vi "Create_Trajectory_Using_PathfinderDifferential_ORIG.vi"() -> ()   [LabVIEW 2019]
uses:
  <vilib>/Rock Robotics/WPI/ThirdParty/JAS_Junk/JaciPathFinderLib/VIs/Waypoint.ctl
  <vilib>/Rock Robotics/WPI/ThirdParty/JAS_Junk/TrajLib/TRAJ_STATE.ctl
  <vilib>/Rock Robotics/WPI/ThirdParty/JAS_Junk/TrajLib/POSE2D.ctl
  <vilib>/Rock Robotics/WPI/ThirdParty/JAS_Junk/TrajLib/TRANSLATION2D.ctl
  <vilib>/Rock Robotics/WPI/ThirdParty/JAS_Junk/TrajLib/ROTATION2D.ctl
  <vilib>/Rock Robotics/WPI/ThirdParty/JAS_Junk/TrajLib/UTIL_PATHFINDER_CONFIG.ctl
  <vilib>/Rock Robotics/WPI/ThirdParty/JAS_Junk/TrajLib/DISPLAY_WAYPOINT.ctl
  <vilib>/Rock Robotics/WPI/ThirdParty/JAS_Junk/JaciPathFinderLib/Pathfinder.lvlib
  <vilib>/Rock Robotics/WPI/ThirdParty/JAS_Junk/TrajLib/Trajectory_Library.lvlib
panel:
  in  "End Program":bool
  in  "Tab Control":T1(tab)
  in  "max_velocity":dbl=58.0
  in  "max_acceleration":dbl=65.0
  in  "max_jerk":dbl=70.0
  in  "wheelbase_width":dbl=20.866
  in  "Real max\n speed":dbl=65.0
  out "max speed":dbl
  out "Path \nSpeed > \nMax":bool
  out "Complete,\nReady to \nSave file":bool
  in  "Calculate\nPath":bool
  out "Path calculation error":errorcluster
  in  "sample_count":i32=100000
  in  "Path Results\ndT":dbl=0.02 format="%7.3f"
  in  "?":T2[](array[typedef])=[{"x"=15.0, "y"=105.0, "angle"=-45.0}, {"x"=105.0, "y"=65.0, "angle"=0.0}, {"x"=210.0, "y"=106.0, "angle"=45.0}]
  out "Position":cluster{dbl[], dbl[]}[](graph)
  out "Path Data":cluster{dbl[], dbl[]}[](graph)
  out "Traj States\nSize":i32
  out "Trajectory States":T3[](array[typedef]) {"POSE"."ROTATION"."SIN" format="%13.4f"; "POSE"."ROTATION"."COS" format="%13.4f"; "POSE"."ROTATION"."VALUE" format="%13.4f"; "POSE"."TRANSLATION"."Y" format="%14.3f"; "POSE"."TRANSLATION"."X" format="%14.3f"}
  out "File Saved\nWithout\nError":bool
  in  "Trajectory Type":enum32{"Radio Selection 1", "Radio Selection 2"}(radio)
  out "File Creation\nError":errorcluster
  in  "Trajectory File Comment":string
  in  "Trajectory File Name":path
  in  "CreateCmdList":bool
  # "Create trajectory using \"Jaci's Pathfinder\"  (Display for differential drive robot)"
  # "Instructions:\n----------------  \nThis utility will create a trajectory,, show the data on the various tabs, and optionally write a \"robot relative\" trajectory to a \nfile. To use this utility:\n\n1) Read all of these instructions!\n2) Define the Robot Data. on the \"Robot Data\" tab.\n3) Define the \"Path Definition\" on the \"Define / Create Trajectory\" tab.  These are the beginning and ending positions/headings, and \n     internal positions/headings.\n4) Define the time increment.  0.020 is chosen since that matches the normal robot loop time.\n5) Define \"sample count\".  This is an internal PathFinder variable.  Leaving the value as default should work correctly.  Making \n    the value a little smaller will speed the program up a little.\n6) Press the \"Calculate Path\".  If a good path was calculated it will be displayed on the \"Field Position tab, and the \"Complete, \n    Ready to Save\" indicator will light.  The path can be recalculated many times before performing any other action.\n\nAfter a Path has been calculated, the \"trajectory can be written to a file.  The absolute path is converted to a robot relative \ntrajectory.  To do this:\n1) Enter a comment to be included in the file.  Anything can be entered.\n2) Select the file name.\n3) Select the type of trajectory to save, absolute or relative.\n4) Press \"Create Trajectory File\"  If an error occurs it will be displayed in the File Creation Error indicator.\n\nNotes:\n---------\n- All the robot parameters, path, and field dimensions are in INCHES, and DEGREES.  The resulting trajectory is converted to \n   METERS, and RADIANS to match the rest of this library!\n- The pathfinder path generation logic doesn't account distribution of speed to the left and right wheels.  As a result the \n   maximum speed can be exceeded.If this happens, but Path Speed > Max light will light and Ready to Execute will not \n   light.  Lower the maximum speed in the Robot Data tab and recalulate the path.  (CURRENTLY THIS LOGIC IS NOT COMPLETE.)\n- 2019 playing field size - width: 26 ft 11.25 In = 323.25 in , length: 52 ft 5.25 in = 629.25 in  (I didn't verify this for the 2020 version.)"
  # "ROBOT DATA"
  # "INCHES/SEC"
  # "INCHES/SEC"
  # "INCHES/SEC^2"
  # "INCHES/SEC^3"
  # "Simulated robot wheelbase is: 20.866"
  # "INCHES"
  # "Simulated robot max speed is: 68.266"
  # "PATH DEFINITION"
  # "SEC"
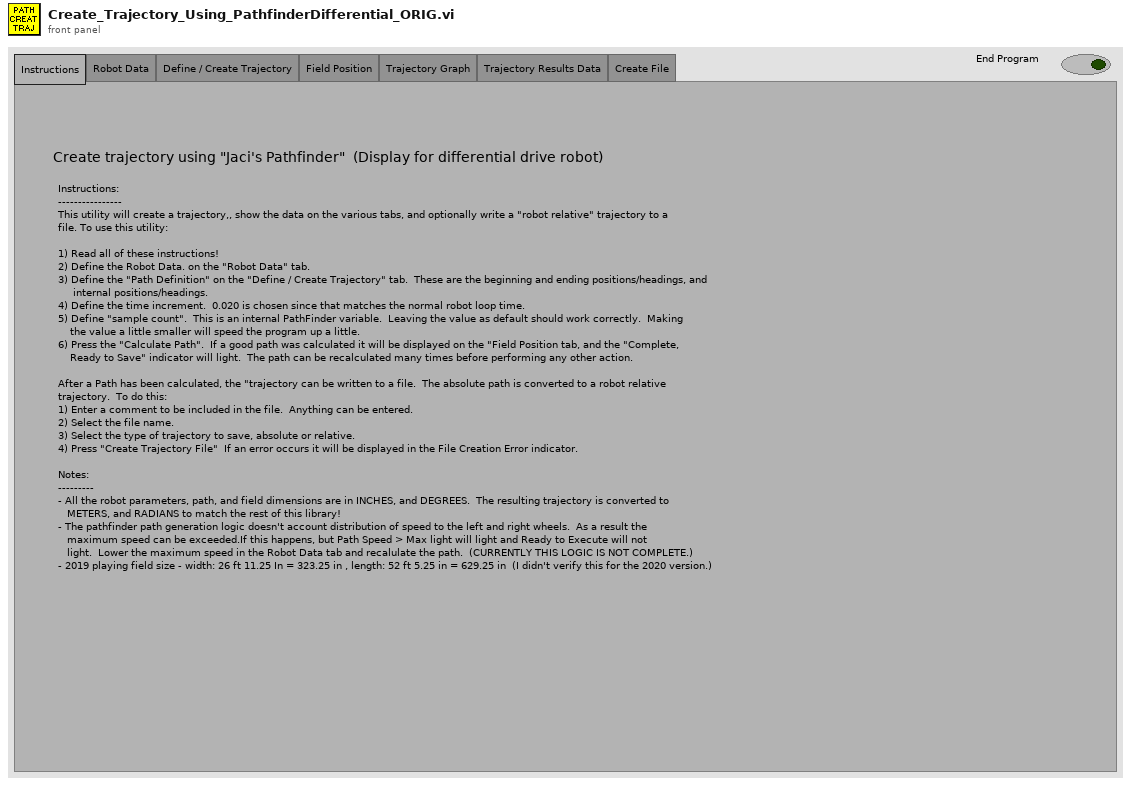
[diagram p1: front panel]
types:
  T1 = enum32{"Instructions", "Robot Data", "Define / Create Trajectory", "Field Position", "Trajectory Graph", "Trajectory Results Data", "Create File"}
  T2 = typedef "Pathfinder.lvlib/Waypoint.ctl" = cluster{"x":dbl, "y":dbl, "angle":dbl}
  T3 = typedef "Trajectory_Library.lvlib/TRAJ_STATE.ctl" = cluster{"TimeSeconds":dbl, "Velocity":dbl, "Acceleration":dbl, "POSE":T4, "Curvature":dbl}
  T4 = typedef "Trajectory_Library.lvlib/POSE2D.ctl" = cluster{"TRANSLATION":T5, "ROTATION":T6}
  T5 = typedef "Trajectory_Library.lvlib/TRANSLATION2D.ctl" = cluster{"X":dbl, "Y":dbl}
  T6 = typedef "Trajectory_Library.lvlib/ROTATION2D.ctl" = cluster{"VALUE":dbl, "COS":dbl, "SIN":dbl}
  T7 = typedef "Trajectory_Library.lvlib/DISPLAY_WAYPOINT.ctl" = cluster{"X":dbl, "Y":dbl, "ANGLE":dbl}
  T8 = typedef "Trajectory_Library.lvlib/UTIL_PATHFINDER_CONFIG.ctl" = cluster{"PathfinderType - 0 tank 1 serve":i32, "PathMaxVelocity - inches per sec":dbl, "MaxAcceleration - inches per sec2":dbl, "MaxJerk--Inches per sec2":dbl, "TimeDelta-Seconds":dbl, "SampleCount":i32, "WheelbaseWidth-inches":dbl, "WheelbaseDepth-inches":dbl, "SwerveType":i32, "ActualMaxVelocity-inches per sec":dbl}
  T9 = typedef "Trajectory_Library.lvlib/TRAJECTORY.ctl" = cluster{"TotalTImeSecs":dbl, "States":T3[]}
  T10 = typedef "Pathfinder.lvlib/Segment.ctl" = cluster{"dt":dbl, "x":dbl, "y":dbl, "position":dbl, "velocity":dbl, "acceleration":dbl, "jerk":dbl, "heading":dbl}
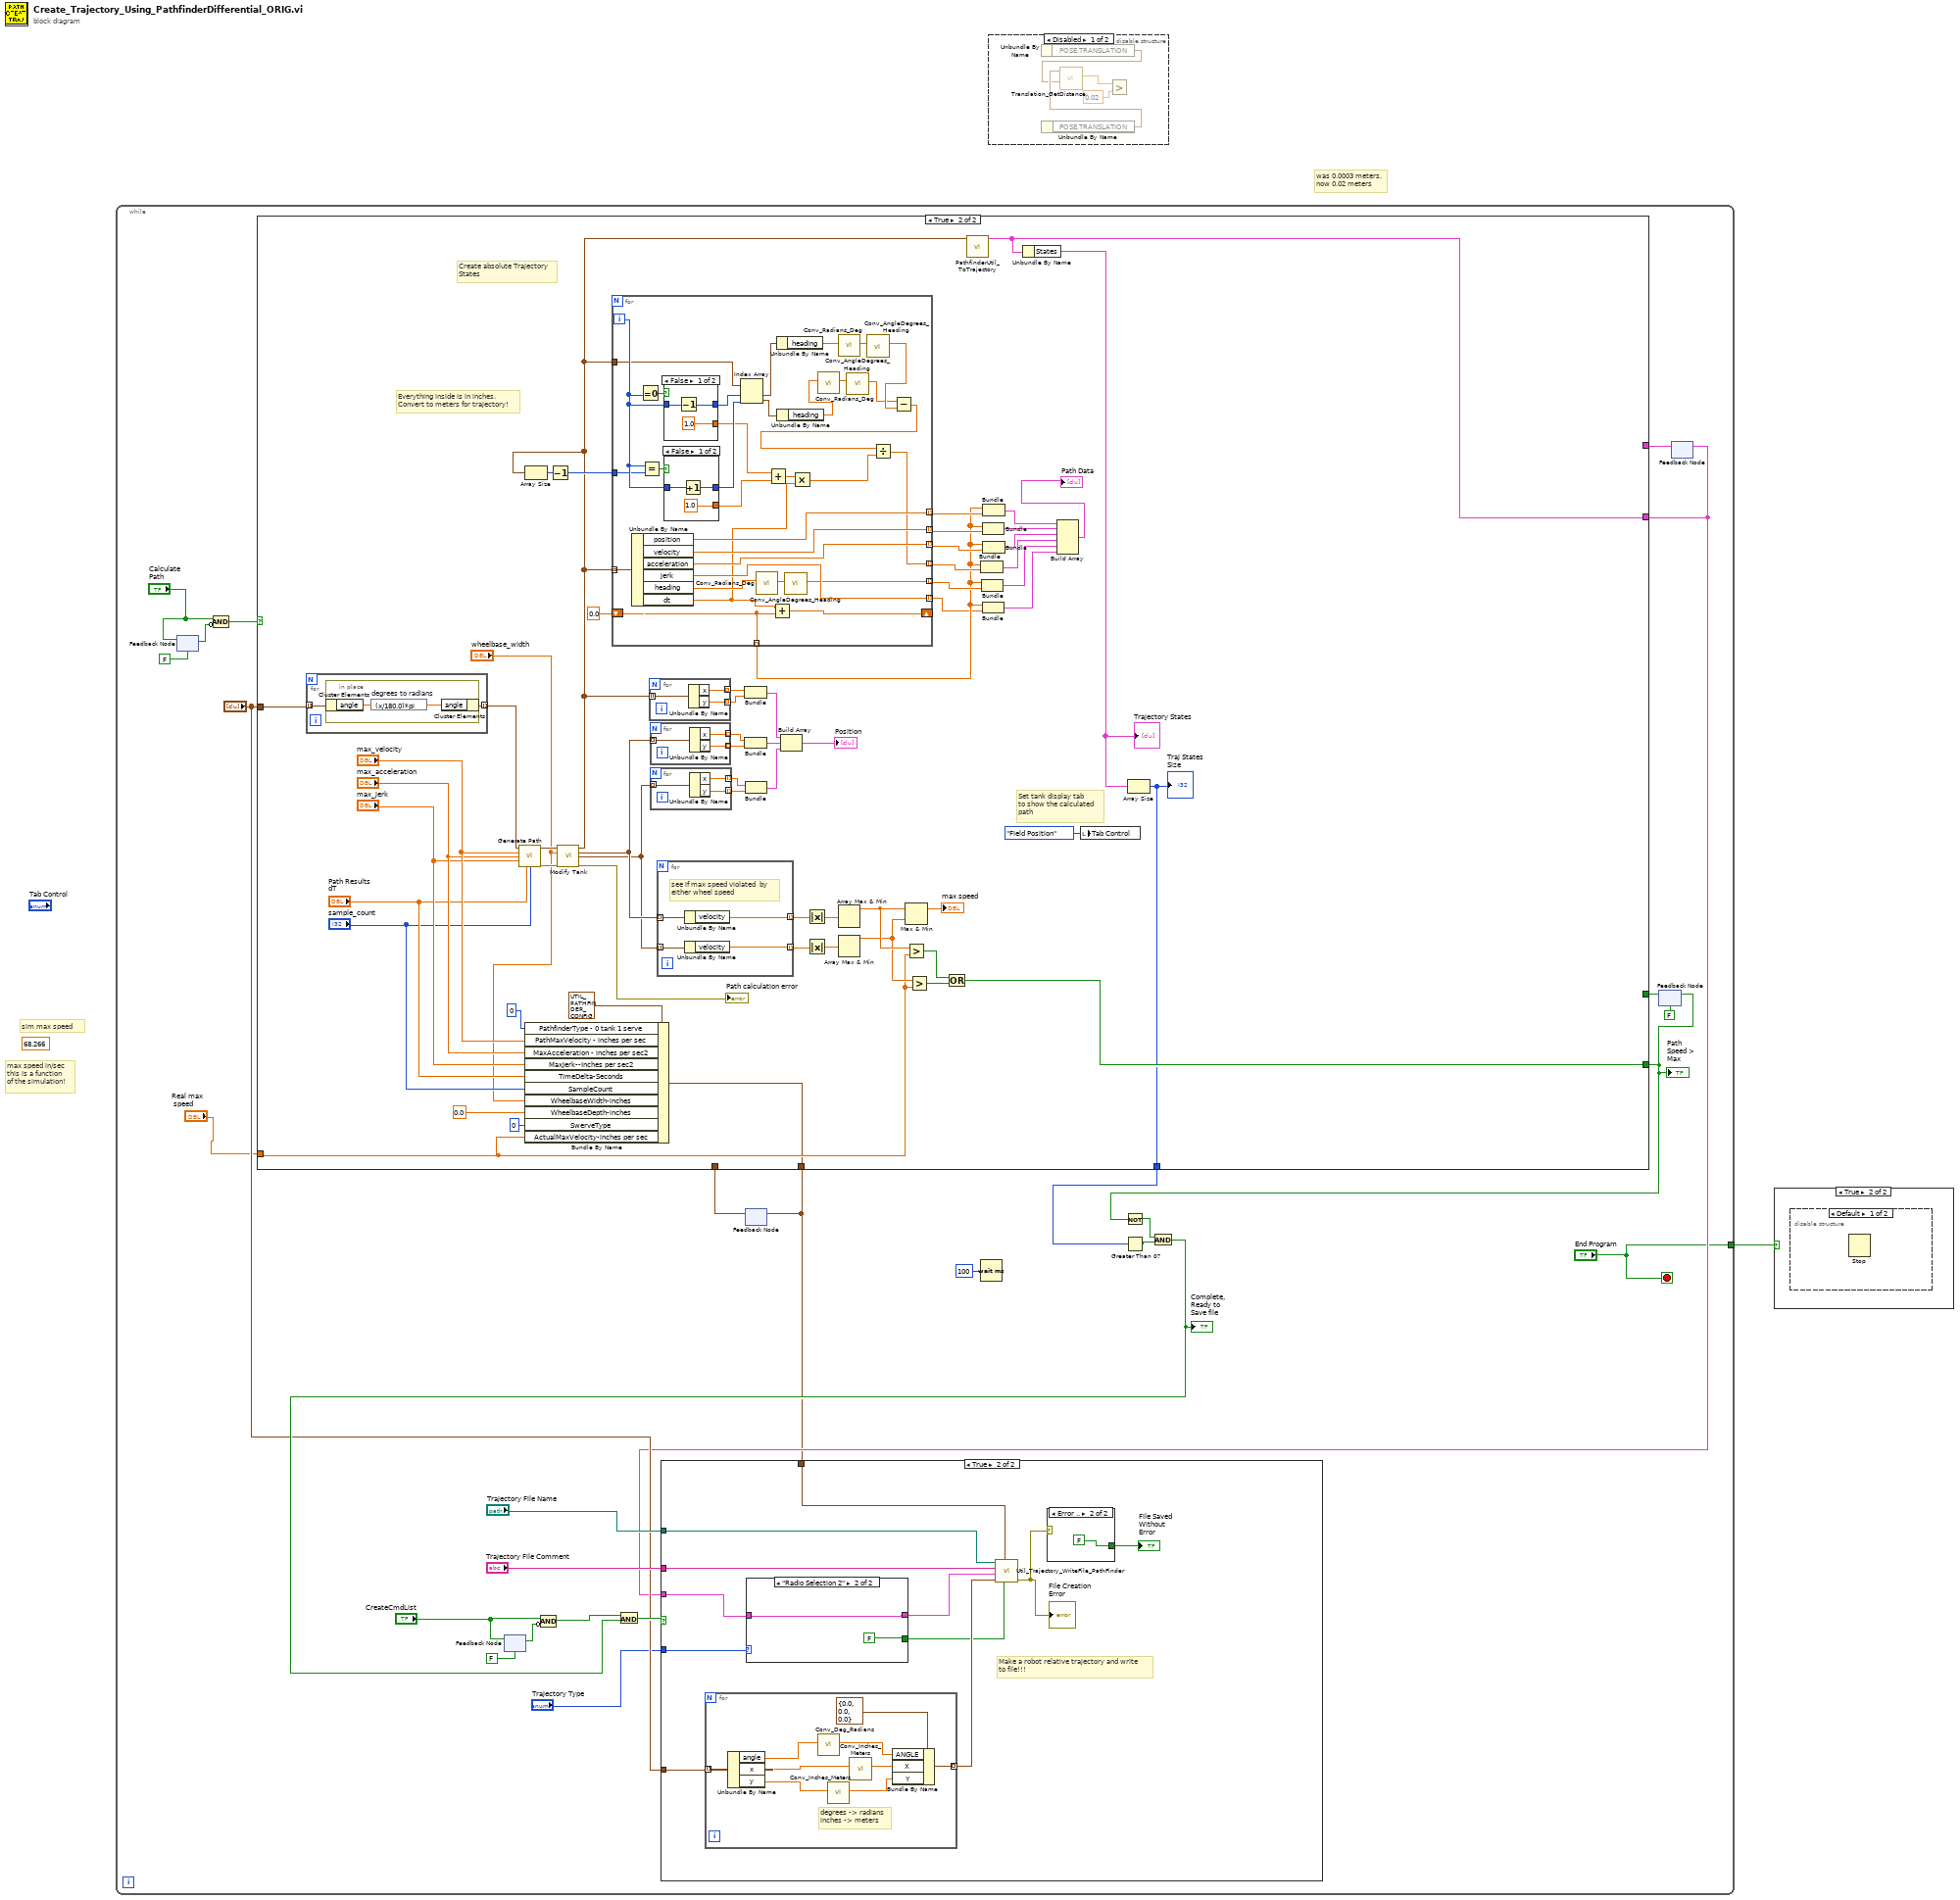
[diagram p0: block diagram]
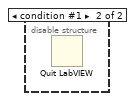
[diagram p3: hidden frame]
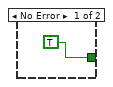
[diagram p6: hidden frame]
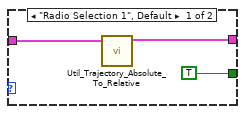
[diagram p7: hidden frame]
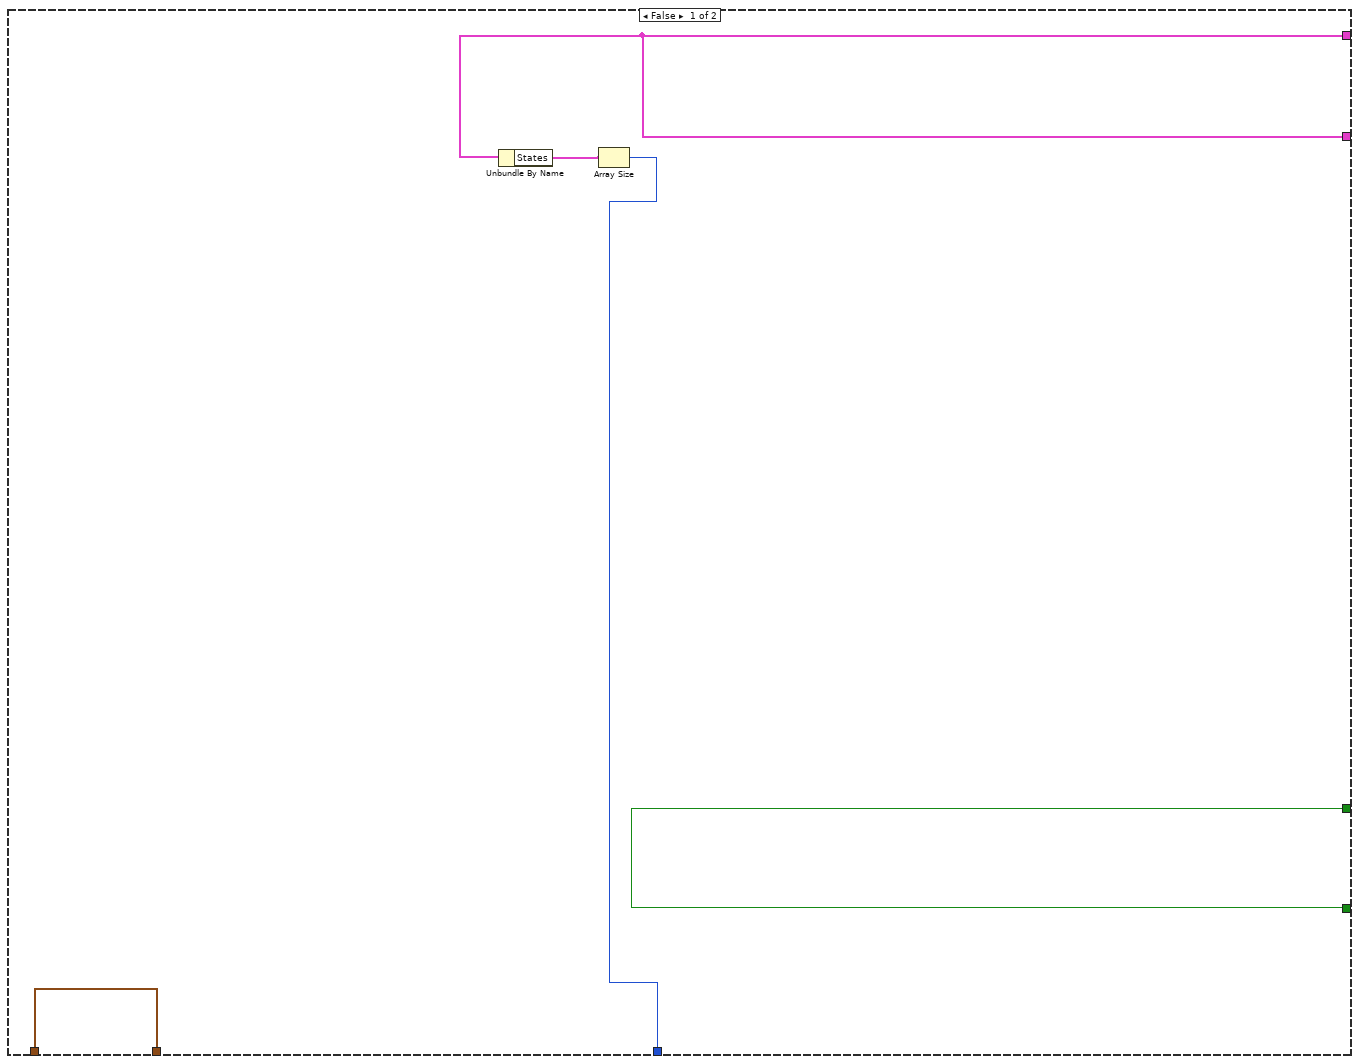
[diagram p8: hidden frame]
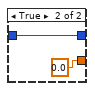
[diagram p9: hidden frame]
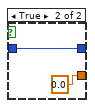
[diagram p10: hidden frame]
diagram:
  (unwired) 68.266 ("x")
  # "was 0.0003 meters.\nnow 0.02 meters"
  # "sim max speed"
  # "max speed in/sec\nthis is a function\nof the simulation!"
  n1 = while {
    tunnel: ["End Program"] -> w1
    stop <- "End Program" stop-if-true
    n2 = feedback #1(FALSE ("CreateCmdList")) -> (w10:bool)
    n3 = feedback-in #1("Calculate\nPath") -> ()
    n4 = Compound Arithmetic op=AND("Calculate\nPath", invert w10) -> (w7:bool)
    n5 = feedback-in #2("CreateCmdList") -> ()
    n6 = feedback #2(FALSE ("CreateCmdList")) -> (w13:bool)
    n7 = Compound Arithmetic op=AND("CreateCmdList", invert w13) -> (w12:bool)
    n8 = feedback #3() -> (w2:T8)  [unwired: 1 in]
    n9 = Wait (ms)(milliseconds to wait=u32 100) -> ()  [unwired: 1 out]
    n10 = feedback #4(FALSE) -> (w26:bool)
    n11 = feedback #5() -> (w22:T9)  [unwired: 1 in]
    n12 = case shown="True" w7 {
      tunnel: "Real max\n speed" -> [_ w65]
      tunnel: [w60 w106] -> w23
      tunnel: w26 -> [w60 _]
      tunnel: "?" -> [_ w105]
      tunnel: [w57 w82] -> w16
      tunnel: w22 -> [w57 _]
      tunnel: [w59 w97] -> w15
      tunnel: [w56 w61] -> w3
      tunnel: w2 -> [w56 _]
      frame False {
        n13 = Unbundle By Name(w57) -> ("States"=w58:T3[])
        n14 = Array Size(array=w58) -> (size(s)=w59:i32)
      }
      frame True {
        # "Everything inside is in inches.\nConvert to meters for trajectory!"
        # "Create absolute Trajectory\nStates"
        # "Set tank display tab\nto show the calculated\npath"
        n15 = for {
          tunnel: w105 -> [w127] mode=indexing
          tunnel: [w126] -> w119 mode=indexing
          n16 = in-place {
            n17 = in-place-cluster #6(w127) -> ("angle"=w129:dbl)
            n18 = expression code="(x/180.0)*pi" "degrees to radians"(w129) -> (w128:dbl)
            n19 = in-place-cluster #6("angle"=w128) -> (w126:T2)
          }
        }
        n20 = call <vilib>:"Generate Path.vi"("path"=w119, "max_velocity"="max_velocity", "max_acceleration"="max_acceleration", "max_jerk"="max_jerk", "dt (.001)"="Path Results\ndT", "sample_count (100000)"="sample_count") -> ("Segments"=w120:T10[], "error out"=w109:errorcluster)  [unwired: 8 in]
        n21 = Bundle By Name(cluster=T8 {"PathfinderType - 0 tank 1 serve"=0, "PathMaxVelocity - inches per sec"=0.0, "MaxAcceleration - inches per sec2"=0.0, "MaxJerk--Inches per sec2"=0.0, "TimeDelta-Seconds"=0.0, "SampleCount"=0, "WheelbaseWidth-inches"=0.0, "WheelbaseDepth-inches"=0.0, "SwerveType"=0, "ActualMaxVelocity-inches per sec"=0.0} ("UTIL_PATHFINDER_CONFIG"), "PathfinderType - 0 tank 1 serve"=0, "PathMaxVelocity - inches per sec"="max_velocity", "MaxAcceleration - inches per sec2"="max_acceleration", "MaxJerk--Inches per sec2"="max_jerk", "TimeDelta-Seconds"="Path Results\ndT", "SampleCount"="sample_count", "WheelbaseWidth-inches"="wheelbase_width", "WheelbaseDepth-inches"=0.0, "SwerveType"=0, "ActualMaxVelocity-inches per sec"=w65) -> (w61:T8)
        n22 = call <vilib>:"Modify Tank.vi"("Original"=w120, "wheelbase_width"="wheelbase_width", "error in"=w109) -> ("original"=w73:T10[], "left"=w104:T10[], "right"=w103:T10[], "error out"=→"Path calculation error":errorcluster)  [unwired: 9 in]
        n23 = Array Size(array=w73) -> (size(s)=w75:i32)
        n24 = Decrement(x=w75) -> (x-1=w74:i32)
        n25 = for {
          tunnel: w73 -> [w170] mode=indexing
          shift-right: [w168] -> _
          shift-left: 0.0 -> [w169]
          tunnel: [w169] -> w78 mode=indexing
          tunnel: [w161] -> w79 mode=indexing
          tunnel: [w167] -> w77 mode=indexing
          tunnel: [w166] -> w87 mode=indexing
          tunnel: [w165] -> w86 mode=indexing
          tunnel: [w164] -> w81 mode=indexing
          tunnel: [w147] -> w80 mode=indexing
          tunnel: w73 -> [w153]
          tunnel: w74 -> [w146]
          i -> [w158]
          n26 = Unbundle By Name(w170) -> ("position"=w164:dbl, "velocity"=w165:dbl, "acceleration"=w166:dbl, "jerk"=w167:dbl, "heading"=w163:dbl, "dt"=w149:dbl)
          n27 = Equal To 0?(x=w158) -> (x = 0?=w160:bool)
          n28 = Equal?(x=w158, y=w146) -> (x = y?=w159:bool)
          n29 = case shown="False" w160 {
            tunnel: w158 -> [w178 w179]
            tunnel: [1.0 0.0] -> w150
            tunnel: [w176 w179] -> w155
            frame False {
              n30 = Decrement(x=w178) -> (x-1=w176:i32)
            }
            frame True {
            }
          }
          n31 = case shown="False" w159 {
            tunnel: [1.0 0.0] -> w151
            tunnel: w158 -> [w172 w174]
            tunnel: [w171 w174] -> w154
            frame False {
              n32 = Increment(x=w172) -> (x+1=w171:i32)
            }
            frame True {
            }
          }
          n33 = Index Array(array=w153, index #1=w155, index #2=w154) -> (element #1=w157:T10, element #2=w156:T10)
          n34 = call <vilib>:"Conv_Radians_Deg.vi"("Radians"=w163) -> ("Degrees"=w162:dbl)  [unwired: 10 in]
          n35 = Add(x=w150, y=w151) -> (x+y=w152:dbl)
          n36 = Add(x=w149, y=w169) -> (x+y=w168:dbl)
          n37 = Unbundle By Name(w157) -> ("heading"=w143:dbl)
          n38 = Unbundle By Name(w156) -> ("heading"=w141:dbl)
          n39 = call <vilib>:"Conv_AngleDegrees_Heading.vi"("Degrees"=w162) -> ("Heading Degrees"=w161:dbl)  [unwired: 10 in]
          n40 = Multiply(x=w152, y=w149) -> (x*y=w148:dbl)
          n41 = call <vilib>:"Conv_Radians_Deg.vi"("Radians"=w141) -> ("Degrees"=w140:dbl)  [unwired: 10 in]
          n42 = call <vilib>:"Conv_Radians_Deg.vi"("Radians"=w143) -> ("Degrees"=w144:dbl)  [unwired: 10 in]
          n43 = call <vilib>:"Conv_AngleDegrees_Heading.vi"("Degrees"=w140) -> ("Heading Degrees"=w139:dbl)  [unwired: 10 in]
          n44 = call <vilib>:"Conv_AngleDegrees_Heading.vi"("Degrees"=w144) -> ("Heading Degrees"=w142:dbl)  [unwired: 10 in]
          n45 = Subtract(x=w139, y=w142) -> (x-y=w145:dbl)
          n46 = Divide(x=w145, y=w148) -> (x/y=w147:dbl)
        }
        n47 = for {
          tunnel: w73 -> [w132] mode=indexing
          tunnel: [w131] -> w116 mode=indexing
          tunnel: [w130] -> w117 mode=indexing
          n48 = Unbundle By Name(w132) -> ("x"=w131:dbl, "y"=w130:dbl)
        }
        n49 = for {
          tunnel: w104 -> [w138] mode=indexing
          tunnel: [w137] -> w110 mode=indexing
          tunnel: [w136] -> w111 mode=indexing
          n50 = Unbundle By Name(w138) -> ("x"=w137:dbl, "y"=w136:dbl)
        }
        n51 = for {
          tunnel: w103 -> [w135] mode=indexing
          tunnel: [w134] -> w112 mode=indexing
          tunnel: [w133] -> w113 mode=indexing
          n52 = Unbundle By Name(w135) -> ("x"=w134:dbl, "y"=w133:dbl)
        }
        n53 = for {
          tunnel: w104 -> [w125] mode=indexing
          tunnel: w103 -> [w124] mode=indexing
          tunnel: [w123] -> w102 mode=indexing
          tunnel: [w122] -> w100 mode=indexing
          # "see if max speed violated  by\neither wheel speed"
          n54 = Unbundle By Name(w125) -> ("velocity"=w123:dbl)
          n55 = Unbundle By Name(w124) -> ("velocity"=w122:dbl)
        }
        n56 = Bundle(w116, w117) -> (w118:cluster{dbl[], dbl[]})  [unwired: 1 in]
        n57 = Bundle(w110, w111) -> (w115:cluster{dbl[], dbl[]})  [unwired: 1 in]
        n58 = Bundle(w112, w113) -> (w114:cluster{dbl[], dbl[]})  [unwired: 1 in]
        n59 = Build Array(w118, w115, w114) -> (→"Position":cluster{dbl[], dbl[]}[])
        n60 = Absolute Value(x=w102) -> (abs(x)=w101:dbl[])
        n61 = Absolute Value(x=w100) -> (abs(x)=w99:dbl[])
        n62 = Array Max & Min(array=w101) -> (max value=w96:dbl)  [unwired: 3 out]
        n63 = Array Max & Min(array=w99) -> (max value=w95:dbl)  [unwired: 3 out]
        n64 = Max & Min(x=w96, y=w95) -> (max(x,y)=→"max speed":dbl)  [unwired: 1 out]
        n65 = Greater?(x=w96, y=w65) -> (0:w107:bool)
        n66 = Greater?(x=w95, y=w65) -> (0:w98:bool)
        n67 = Compound Arithmetic op=OR(w107, w98) -> (w106:bool)
        n68 = call <vilib>:"PathfinderUtil_ToTrajectory.vi"("Pathfinder Path"=w73) -> ("TRAJECTORY"=w82:T9)  [unwired: 10 in]
        n69 = Bundle(w78, w80) -> (w90:cluster{dbl[], dbl[]})  [unwired: 1 in]
        n70 = Bundle(w78, w79) -> (w89:cluster{dbl[], dbl[]})  [unwired: 1 in]
        n71 = Bundle(w78, w86) -> (w92:cluster{dbl[], dbl[]})  [unwired: 1 in]
        n72 = Bundle(w78, w77) -> (w76:cluster{dbl[], dbl[]})  [unwired: 1 in]
        n73 = Bundle(w78, w81) -> (w93:cluster{dbl[], dbl[]})  [unwired: 1 in]
        n74 = Bundle(w78, w87) -> (w91:cluster{dbl[], dbl[]})  [unwired: 1 in]
        n75 = Unbundle By Name(w82) -> ("States"=w84:T3[])
        "Trajectory States" <- w84
        n76 = Build Array(w93, w92, w91, w90, w89, w76) -> (→"Path Data":cluster{dbl[], dbl[]}[])
        n77 = local write "Tab Control"(T1."Field Position" ("Tab Control")) -> ()
        n78 = Array Size(array=w84) -> (size(s)=w97:i32)
        "Traj States\nSize" <- w97
      }
    }
    "Path \nSpeed > \nMax" <- w23
    n79 = feedback-in #3(w3) -> ()
    n80 = Not(x=w23) -> (.not. x?=w24:bool)
    n81 = Greater Than 0?(x=w15) -> (x > 0?=w25:bool)
    n82 = And(x=w24, y=w25) -> (x .and. y?=w18:bool)
    "Complete,\nReady to \nSave file" <- w18
    n83 = And(x=w12, y=w18) -> (x .and. y?=w19:bool)
    n84 = case shown="True" w19 {
      tunnel: "Trajectory File Name" -> [_ w39]
      tunnel: "Trajectory File Comment" -> [_ w38]
      tunnel: w16 -> [_ w34]
      tunnel: "?" -> [_ w37]
      tunnel: "Trajectory Type" -> [_ w33]
      tunnel: w3 -> [_ w29]
      frame False {
      }
      frame True {
        # "Make a robot relative trajectory and write\nto file!!!"
        n85 = for {
          tunnel: w37 -> [w55] mode=indexing
          tunnel: [w54] -> w36 mode=indexing
          # "degrees -> radians\ninches -> meters"
          n86 = Unbundle By Name(w55) -> ("angle"=w48:dbl, "x"=w53:dbl, "y"=w51:dbl)
          n87 = call <vilib>:"Conv_Deg_Radians.vi"("Degress"=w48) -> ("Radians"=w49:dbl)  [unwired: 10 in]
          n88 = call <vilib>:"Conv_Inches_Meters.vi"("INCH"=w51) -> ("Meters"=w50:dbl)  [unwired: 10 in]
          n89 = call <vilib>:"Conv_Inches_Meters.vi"("INCH"=w53) -> ("Meters"=w52:dbl)  [unwired: 10 in]
          n90 = Bundle By Name(cluster=T7 {"X"=0.0, "Y"=0.0, "ANGLE"=0.0} ("UTIL_WAYPOINT"), "ANGLE"=w49, "X"=w52, "Y"=w50) -> (w54:T7)
        }
        n91 = case shown="\"Radio Selection 2\"" w33 {
          tunnel: w34 -> [w44 w46]
          tunnel: [w43 w46] -> w35
          tunnel: [TRUE FALSE] -> w30
          frame "Radio Selection 1", Default {
            n92 = call <vilib>:"Util_Trajectory_Absolute_To_Relative.vi"("absTRAJECTORY"=w44) -> ("outputRelativeTRAJECTORY"=w43:T9)  [unwired: 10 in]
          }
          frame "Radio Selection 2" {
          }
        }
        n93 = call <vilib>:"Util_Trajectory_WriteFile_PathFinder.vi"("Trajectory Is Relative"=w30, "UTIL_PATHFINDER_CONFIG"=w29, "UtilityWayPoints"=w36, "TRAJECTORY"=w35, "Comment"=w38, "Trajectory File Name"=w39) -> ("error out"=w32:errorcluster)  [unwired: 5 in]
        "File Creation\nError" <- w32
        n94 = case shown="Error .." w32 {
          tunnel: [TRUE ("File Saved\nWithout\nError") FALSE ("File Saved\nWithout\nError")] -> w31
          frame No Error {
          }
          frame Error {
          }
        }
        "File Saved\nWithout\nError" <- w31
      }
    }
    n95 = feedback-in #4(w23) -> ()
    n96 = feedback-in #5(w16) -> ()
  }
  n97 = disable-structure shown="Disabled" {
    frame Disabled {
      n98 = Unbundle By Name() -> ("POSE.TRANSLATION"=w184:T5)  [unwired: 1 in]
      n99 = Unbundle By Name() -> ("POSE.TRANSLATION"=w185:T5)  [unwired: 1 in]
      n100 = call <vilib>:"Translation_GetDistance.vi"("other Translation"=w184, "In Translation"=w185) -> ("Distance"=w183:dbl)  [unwired: 9 in]
      n101 = Greater?(x=w183, y=0.02) -> (0:w181:bool)
    }
    frame Enabled {
    }
  }
  n102 = case shown="True" w1 {
    frame False {
    }
    frame True {
      n103 = disable-structure shown="Default" {
        frame condition #0 (active) {
          n104 = Stop() -> ()  [unwired: 1 in]
        }
        frame condition #1 {
          n105 = Quit LabVIEW() -> ()  [unwired: 1 in]
        }
      }
    }
  }
